vi "get_last_minmax.vi"(0 "max_min_array":T1(array[cluster])) -> (1 "max_vector":dbl[](array[numeric]), 2 "min_vector":dbl[](array[numeric]), 3 "distance":dbl)   [LabVIEW 2011]
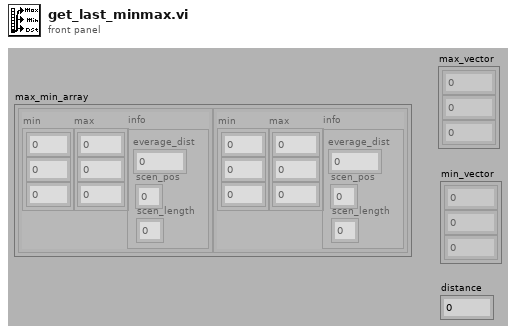
[diagram p1: front panel]
types:
  T1 = cluster{"min":dbl[], "max":dbl[], "info":cluster{"everage_dist":dbl, "scen_pos":u16, "scen_length":u16}}[]
  T2 = cluster{"min":dbl[], "max":dbl[], "info":cluster{"everage_dist":dbl, "scen_pos":u16, "scen_length":u16}}
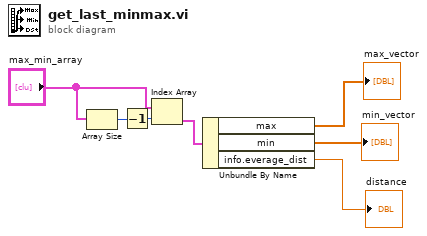
[diagram p0: block diagram]
diagram:
  n1 = Array Size(array="max_min_array") -> (size(s)=w7:i32)
  n2 = Decrement(x=w7) -> (x-1=w6:i32)
  n3 = Index Array(array="max_min_array", index=w6) -> (element=w5:T2)
  n4 = Unbundle By Name(w5) -> ("max"=→"max_vector":dbl[], "min"=→"min_vector":dbl[], "info.everage_dist"=→"distance":dbl)
